vi "Wait dialog.vi"(8 "error in (no error)":errorcluster, 10 "Time":dbl, 11 "String in":refnum<vi>) -> (0 "error out":errorcluster)   [LabVIEW 2019]
doc: "Calculates ETA for a dialog"
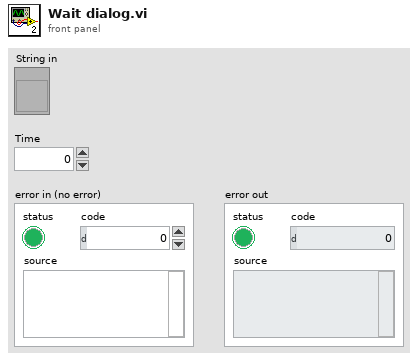
[diagram p1: front panel]
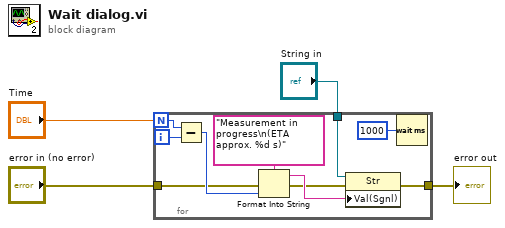
[diagram p0: block diagram]
diagram:
  n1 = for {
    N: "Time" -> [w14]
    tunnel: [w8] -> w2
    tunnel: "error in (no error)" -> [w7]
    tunnel: "String in" -> [w5]
    i -> [w13]
    n2 = Subtract(x=w14, y=w13) -> (x-y=w12:i32)
    n3 = Format Into String(format string="Measurement in progress\n(ETA approx. %d s)", error in=w7, w12) -> (resulting string=w11:string, error out=w9:errorcluster)  [unwired: 1 in]
    n4 = property on="Property Node" class="Str"(reference=w5, error in=w9, "Val(Sgnl)"=w11) -> (error out=w8:errorcluster)  [unwired: 1 out]
    n5 = Wait (ms)(milliseconds to wait=u32 1000) -> ()  [unwired: 1 out]
  }
  "error out" <- w2
